vi "Read Measurement.vi"   [LabVIEW 2022 SP3, in "Agilent N934X Series.lvlib"]
doc: "This is a poly VI for read measurement VIs."
uses:
  <instrlib>/Agilent N934X Series/Agilent N934X Series.lvlib
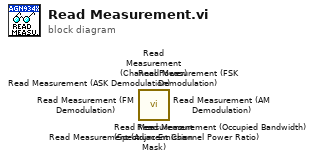
[diagram p0: block diagram]
diagram:
  n1 = call <instrlib>:"Read Measurement (Spectrum Emission Mask).vi"() -> ()  [unwired: 13 in, 3 out]
  n2 = call <instrlib>:"Read Measurement (FSK Demodulation).vi"() -> ()  [unwired: 9 in, 7 out]
  n3 = call <instrlib>:"Read Measurement (FM Demodulation).vi"() -> ()  [unwired: 8 in, 8 out]
  n4 = call <instrlib>:"Read Measurement (AM Demodulation).vi"() -> ()  [unwired: 8 in, 8 out]
  n5 = call <instrlib>:"Read Measurement (ASK Demodulation).vi"() -> ()  [unwired: 9 in, 7 out]
  n6 = call <instrlib>:"Read Measurement (Channel Power).vi"() -> ()  [unwired: 12 in, 4 out]
  n7 = call <instrlib>:"Read Measurement (Occupied Bandwidth).vi"() -> ()  [unwired: 12 in, 4 out]
  n8 = call <instrlib>:"Read Measurement (Adjacent Channel Power Ratio).vi"() -> ()  [unwired: 9 in, 7 out]
